vi "Rig_Name.vi"(0 "Post Process":T1) -> (1 "Rig Setup before dash":string, 2 "Hard Disk name":string)   [LabVIEW 2010]
uses:
  Controls/Post_Process.ctl
  Globals/Preference_global.vi
  Globals/Meas_global.vi
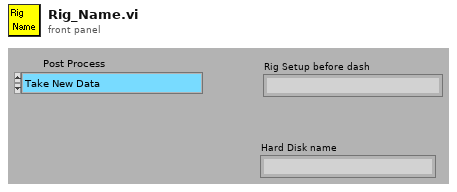
[diagram p1: front panel]
types:
  T1 = typedef "Post_Process.ctl" = enum16{"Take New Data", "Post Process Raw Data File"}
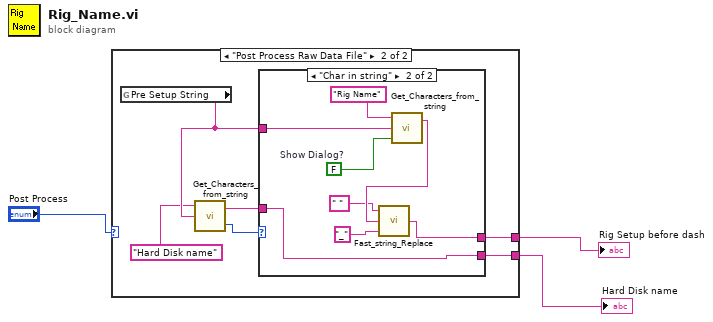
[diagram p0: block diagram]
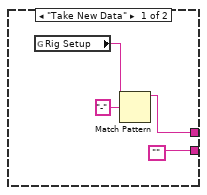
[diagram p2: hidden frame]
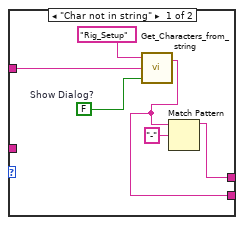
[diagram p3: hidden frame]
diagram:
  n1 = case shown="\"Post Process Raw Data File\"" "Post Process" {
    tunnel: [w4 w13] -> w2
    tunnel: ["" w8] -> w3
    frame "Take New Data" {
      n2 = global read "Preference_global.vi" "Rig Setup"() -> (w5:string)
      n3 = Match Pattern(string=w5, regular expression="-") -> (before substring=w4:string)  [unwired: 4 out]
    }
    frame "Post Process Raw Data File" {
      n4 = global read "Meas_global.vi" "Pre Setup String"() -> (w12:string)
      n5 = call "Get_Characters_from_string.vi"("Input string"=w12, "Variable name"="Hard Disk name") -> ("Status"=w10:enum16{"Char in string", "Char not in string"}, "Value"=w9:string)  [unwired: 1 in]
      n6 = case shown="\"Char in string\"" w10 {
        tunnel: [w15 w20] -> w13
        tunnel: w12 -> [w18 w26]
        tunnel: w9 -> [_ w24]
        tunnel: [w14 w24] -> w8
        frame "Char not in string" {
          w17 = FALSE  # Show Dialog?
          n7 = call "Get_Characters_from_string.vi"("Show Dialog?"=w17, "Input string"=w18, "Variable name"="Rig_Setup") -> ("Value"=w14:string)  [unwired: 1 out]
          n8 = Match Pattern(string=w14, regular expression="-") -> (before substring=w15:string)  [unwired: 4 out]
        }
        frame "Char in string" {
          w25 = FALSE  # Show Dialog?
          n9 = call "Get_Characters_from_string.vi"("Show Dialog?"=w25, "Input string"=w26, "Variable name"="Rig Name") -> ("Value"=w23:string)  [unwired: 1 out]
          n10 = call "Fast_string_Replace.vi"("Replace match with:"="_", "Input String"=w23, "regular expression"=" ") -> ("Output String"=w20:string)  [unwired: 2 out]
        }
      }
    }
  }
  "Hard Disk name" <- w3
  "Rig Setup before dash" <- w2
